vi "AuMT8852B Inquiry Timeout.vi"(5 "Timeout (1)":i32=1, 7 "Set/Get (Set)":enum16{"Set", "Get"}(ring), 8 "error in (no error)":errorcluster, 11 "VISA session":refnum<visa-resource-name>) -> (0 "error out":errorcluster, 2 "error code":i32, 3 "VISA session out":refnum<visa-resource-name>, 4 "Timeout out":i32=1)   [LabVIEW 2017]
doc: "Anritsu MT8852B Bluetooth Tester\n\nMaximum period of time for which the inquiry will run.\n\nINPUTS\nSet/Get - whether the value is being sent to or retrieved from the instrument.\nTimeout - timeout to send to the instrument (in multiples of 1.28 ms).\n\nOUTPUTS\nTimeout out - current timeout stored in the instrument."
uses:
  <instrlib>/aumt8852B/General/Utilities/MT8850 Attribute ID.ctl
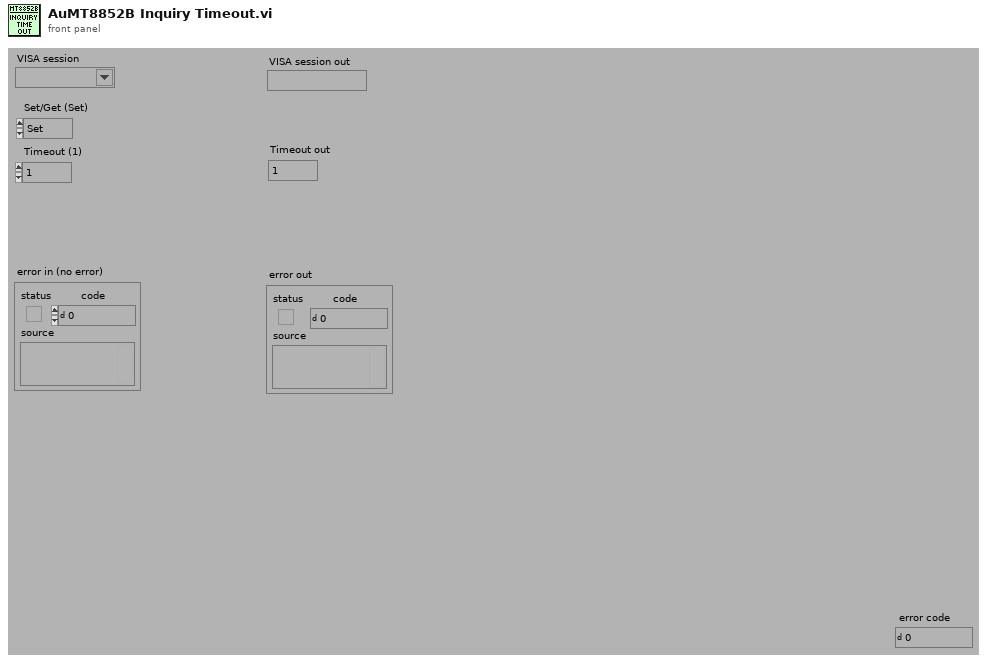
[diagram p1: front panel]
types:
  T1 = typedef "MT8850 Attribute ID.ctl" = enum16{"Operation mode", "Selected script", "EUT address source", "EUT Address", "EUT HCI RS232 Baud Rate", "Tester GPIB Address", "Tester RS232 Baud Rate", "Tester Bluetooth Address", "Tester Contrast", "Tester Key Click On", "Tester Modulation Index", "Tester Poll-Null Mode", "Tester Power Range", "Tester RS232 Mode", "Beep on Illegal Entry", "Display User Text", "User Text", "Calibration TX Modulation DAC", "Calibration RX Channel", "Calibration TX Channel", "Calibration TX Power", "Calibration Use TX Table", "Inquiry Request User-friendly Name", "Inquiry Number of Responses", "Inquiry Timeout", "Script Frequency Display", "Script Loop Count", "Script Loop Continuously", "Script Loop Stop on Fail", "Link timeout", "Page timeout", "Filter bandwidth", "SCO air code", "SCO bit position", "SCO input code", "SCO input data", "SCO input sample size", "SCO loopback mode", "SCO packet type", "SCO tone generator", "Tester page scan repetition mode", "Tester follow test mode", "Tester authentication state", "Tester authentication pin code", "Tester authentication pin length"}
  T2 = typedef "Attribute Status.ctl" = enum16{"No I/O needed", "I/O needed"}
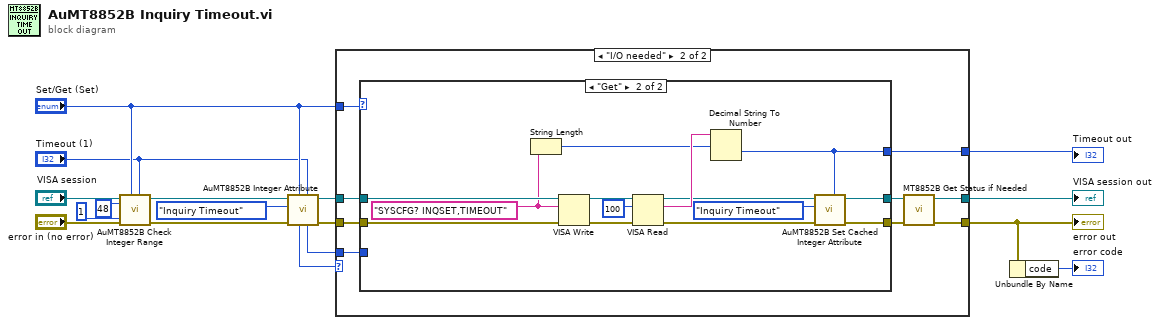
[diagram p0: block diagram]
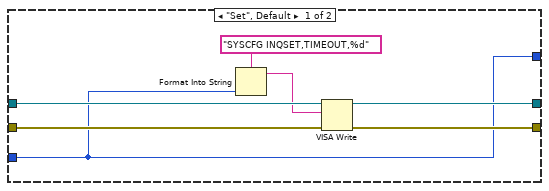
[diagram p3: hidden frame]
diagram:
  n1 = call <instrlib>:"AuMT8852B Check Integer Range.vi"("Value (0)"="Timeout (1)", "Set/Get (Set)"="Set/Get (Set)", "error in (no error)"="error in (no error)", "Lower limit (-1)"=1, "Upper limit (1)"=48, "VISA session"="VISA session") -> ("error out"=w8:errorcluster, "VISA session out"=w9:refnum<visa-resource-name>)  [unwired: 4 in]
  n2 = call <instrlib>:"AuMT8852B Integer Attribute.vi"("Value (0)"="Timeout (1)", "Set/Get (Set)"="Set/Get (Set)", "error in (no error)"=w8, "Attribute ID"=MT8850_Attribute_ID."Inquiry Timeout", "VISA session"=w9) -> ("error out"=w13:errorcluster, "VISA session out"=w14:refnum<visa-resource-name>, "Value out"=w16:i32, "Status"=w12:T2)  [unwired: 3 in]
  n3 = case shown="\"I/O needed\"" w12 {
    tunnel: w16 -> [w18 w27]
    tunnel: [w19 w23] -> w2
    tunnel: [w20 w24] -> w15
    tunnel: w14 -> [w20 w29]
    tunnel: w13 -> [w19 w28]
    tunnel: "Set/Get (Set)" -> [_ w22]
    tunnel: [w18 w21] -> w4
    frame "No I/O needed", Default {
    }
    frame "I/O needed" {
      n4 = case shown="\"Get\"" w22 {
        tunnel: w29 -> [w36 w43]
        tunnel: w28 -> [w35 w42]
        tunnel: w27 -> [w30 _]
        tunnel: [w34 w40] -> w26
        tunnel: [w33 w41] -> w25
        tunnel: [w30 w37] -> w21
        frame "Set", Default {
          n5 = Format Into String(format string="SYSCFG INQSET,TIMEOUT,%d" ("Format String"), w30) -> (resulting string=w31:string)  [unwired: 2 in, 1 out]
          n6 = VISA Write(VISA resource name=w36, write buffer=w31, error in (no error)=w35) -> (VISA resource name out=w34:refnum<visa-resource-name>, error out=w33:errorcluster)  [unwired: 1 out]
        }
        frame "Get" {
          w38 = "SYSCFG? INQSET,TIMEOUT" ("write buffer (\"\")")
          n7 = String Length(string=w38) -> (length=w39:i32)
          n8 = VISA Write(VISA resource name=w43, write buffer=w38, error in (no error)=w42) -> (VISA resource name out=w44:refnum<visa-resource-name>, error out=w46:errorcluster)  [unwired: 1 out]
          n9 = VISA Read(VISA resource name=w44, byte count=u32 100 ("byte count (0)"), error in (no error)=w46) -> (VISA resource name out=w47:refnum<visa-resource-name>, read buffer=w50:string, error out=w48:errorcluster)  [unwired: 1 out]
          n10 = Decimal String To Number(string=w50, offset=w39) -> (number=w37:i32)  [unwired: 1 in, 1 out]
          n11 = call <instrlib>:"AuMT8852B Set Cached Integer Attribute.vi"("Value (0)"=w37, "error in (no error)"=w48, "Attribute ID"=MT8850_Attribute_ID."Inquiry Timeout", "VISA session"=w47) -> ("error out"=w41:errorcluster, "VISA session out"=w40:refnum<visa-resource-name>)  [unwired: 6 in]
        }
      }
      n12 = call <instrlib>:"MT8852B Get Status if Needed.vi"("error in (no error)"=w25, "VISA session"=w26) -> ("error out"=w23:errorcluster, "VISA session out"=w24:refnum<visa-resource-name>)  [unwired: 8 in]
    }
  }
  "error out" <- w2
  "VISA session out" <- w15
  "Timeout out" <- w4
  n13 = Unbundle By Name(w2) -> ("code"=→"error code":i32)
